vi "Main_006.vi"() -> ()   [LabVIEW 2025]
uses:
  Utility/Universal Utility/TypeDefs_Utility/Cluster_Row-Column.ctl
  9e3f57c0-2ef8-4495-8287-c6a42a5fb955.vi
  Utility/Universal Utility/TypeDefs_Utility/ENUM_4 Directions U-D-L-R.ctl
  Utility/Universal Utility/TypeDefs_Utility/ENUM_8 Directions U-D-L-R.ctl
panel:
  out "MATCH":bool
  in  "Select Data":enum32{"Example", "Puzzle"}(tab)
  in  "EX Target":u64=2640
  in  "Example Input":u64=10
  in  "Puzzle Input":u64=100
  in  "Puzzle Target":u64=2516415
  out "Answer":u64
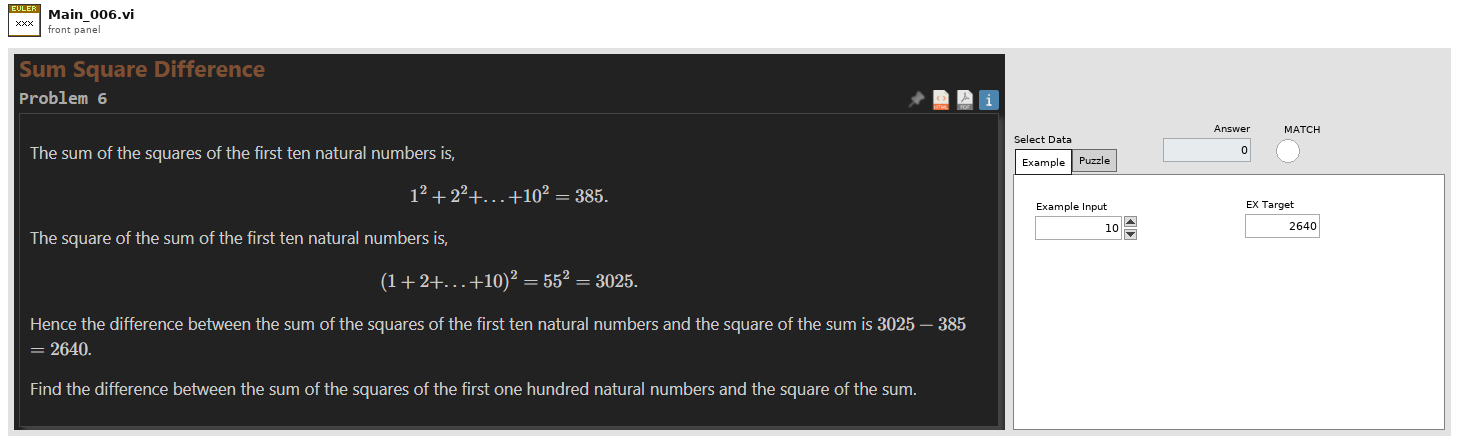
[diagram p1: front panel]
types:
  T1 = typedef "ENUM_8 Directions U-D-L-R.ctl" = enum16{"Up;-1,0", "Up-Right;-1,1", "Right;0,1", "Down-Right;1,1", "Down;1,0", "Down-Left;1,-1", "Left;0,-1", "Up-Left;-1,-1"}
  T2 = typedef "ENUM_4 Directions U-D-L-R.ctl" = enum16{"Up;-1,0", "Right;0,1", "Down;1,0", "Left;0,-1"}
  T3 = typedef "Cluster_Row-Column.ctl" = cluster{"R":i32, "C":i32}
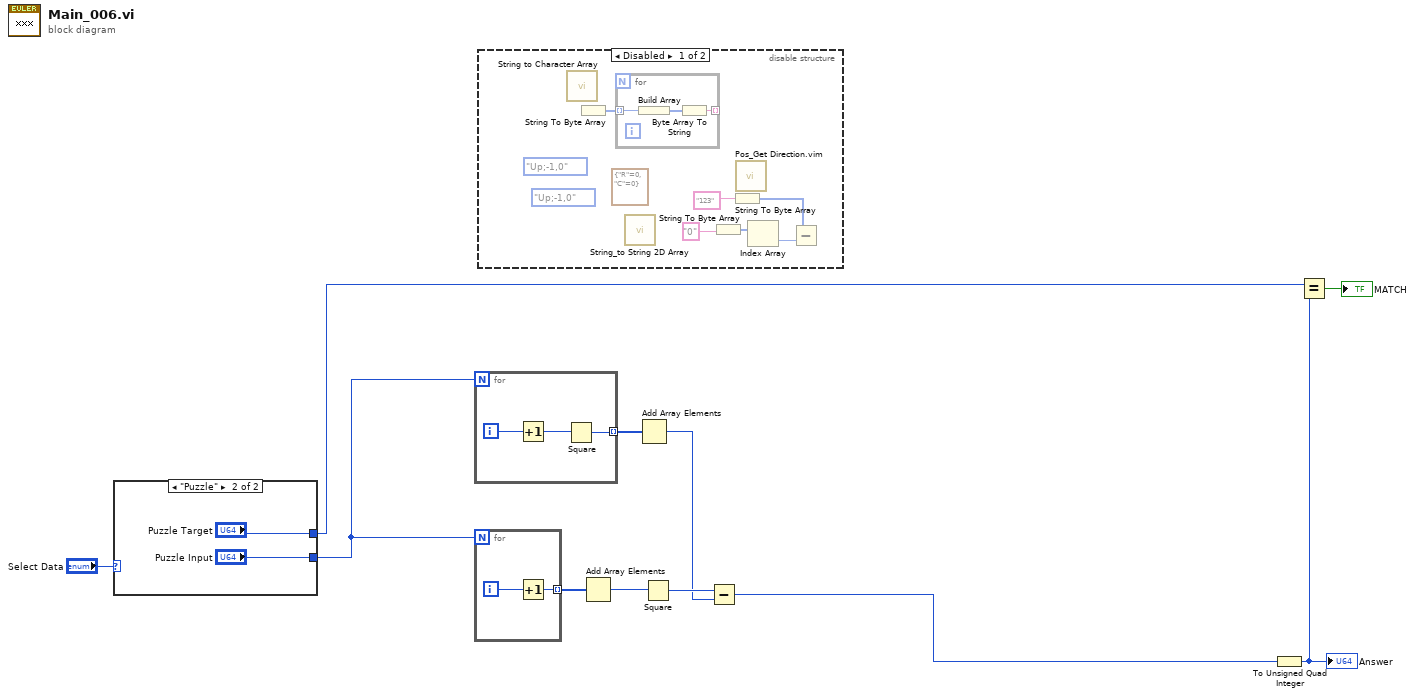
[diagram p0: block diagram]
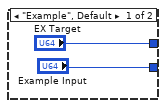
[diagram p2: hidden frame]
diagram:
  n1 = case shown="\"Puzzle\"" "Select Data" {
    tunnel: ["Example Input" "Puzzle Input"] -> w6
    tunnel: ["EX Target" "Puzzle Target"] -> w9
    frame "Example", Default {
    }
    frame "Puzzle" {
    }
  }
  n2 = for {
    N: w6 -> [_]
    tunnel: [w16] -> w7 mode=indexing
    i -> [w18]
    n3 = Increment(x=w18) -> (x+1=w17:i32)
    n4 = Square(x=w17) -> (x^2=w16:i32)
  }
  n5 = for {
    N: w6 -> [_]
    tunnel: [w19] -> w5 mode=indexing
    i -> [w20]
    n6 = Increment(x=w20) -> (x+1=w19:i32)
  }
  n7 = disable-structure shown="Disabled" {
    frame Disabled {
      (unwired) ENUM_8_Directions_U-D-L-R."Up;-1,0" ("Direction 8")
      (unwired) ENUM_4_Directions_U-D-L-R."Up;-1,0" ("Direction")
      (unwired) T3 {"R"=0, "C"=0} ("Position")
      n8 = call "String to Character Array.vi"() -> ()  [unwired: 1 in, 1 out]
      n9 = String To Byte Array() -> (unsigned byte array=w21:u8[])  [unwired: 1 in]
      n10 = for {
        tunnel: w21 -> [w29] mode=indexing
        tunnel: [w27] -> _ mode=indexing
        n11 = Build Array(w29) -> (w28:u8[])
        n12 = Byte Array To String(unsigned byte array=w28) -> (string=w27:string)
      }
      n13 = call "String_to String 2D Array.vi"() -> ()  [unwired: 11 in, 1 out]
      n14 = String To Byte Array(string="0") -> (unsigned byte array=w24:u8[])
      n15 = String To Byte Array(string="123") -> (unsigned byte array=w22:u8[])
      n16 = call "Pos_Get Direction.vim"() -> ()  [unwired: 11 in, 1 out]
      n17 = Index Array(array=w24) -> (element=w23:u8)  [unwired: 1 in]
      n18 = Subtract(x=w22, y=w23) -> ()  [unwired: 1 out]
    }
    frame Enabled {
    }
  }
  n19 = Add Array Elements(numeric array=w5) -> (sum=w2:i32)
  n20 = Add Array Elements(numeric array=w7) -> (sum=w3:i32)
  n21 = Square(x=w2) -> (x^2=w4:i32)
  n22 = Subtract(x=w4, y=w3) -> (x-y=w1:i32)
  n23 = To Unsigned Quad Integer(1:w1) -> (0:w8:u64)
  "Answer" <- w8
  n24 = Equal?(x=w9, y=w8) -> (x = y?=→"MATCH":bool)
